vi "XML - Get relative RT Driver VI path.vi"(7 "Target Type (Windows)":T1, 10 "CD Template":refnum<class "NIVS_CD Template.lvclass">, 11 "Project Name":string) -> (3 "Relative RT Driver VI path":path)   [LabVIEW 2015, in "NIVS_Consolidated_CDW_MetaDataObj.lvclass"]
doc: "Create the relative path for the RT Driver VI inside the Configuration LLB based on the name and execution mode of the new custom device."
uses:
  NIVS_Consolidated_CDW_MetaDataObj.lvclass
  Target Type.ctl
  Template Classes/NIVS_CD Template/NIVS_CD Template.lvclass
  CD Engine lvlib.ctl
  Build Spec Engine.ctl
  Build Spec Engine.vi
  CD Engine lvlib.vi
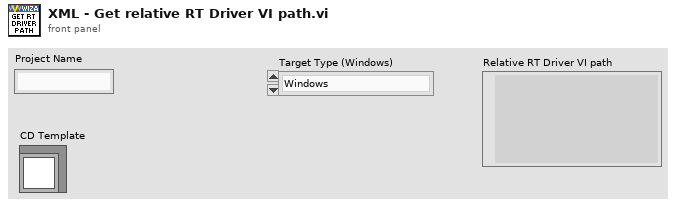
[diagram p1: front panel]
types:
  T1 = typedef "NIVS_Consolidated_CDW_MetaDataObj.lvclass/Target Type.ctl" = enum16{"Windows", "VxWorks", "Pharlap", "Linux 32 ARM", "Linux x64"}
  T2 = typedef "NIVS_Consolidated_CDW_MetaDataObj.lvclass/CD Engine lvlib.ctl" = enum16{"LibraryFileName", "LibraryFolderName", "Engine.FolderName", "Engine.Init.FolderName", "Engine.Run.FolderName", "Engine.Shutdown.FolderName", "Types.FolderName", "Engine.RT Driver VI.TemplatePath", "Engine.RT Driver VI.FileName", "Engine.RTStateVariables.Name", "Engine.RTStateVariables.Name.NoExtension", "Engine.Async.NameExtension", "Engine.Async.TemplateName"}
  T3 = typedef "NIVS_Consolidated_CDW_MetaDataObj.lvclass/Build Spec Engine.ctl" = enum16{"Destinations.LLBWindowsFileName", "Destinations.LLBVxWorksFileName", "Destinations.LLBPharlapFileName", "Destinations.LLBLinuxARMFileName", "Destinations.LLBLinux64FileName"}
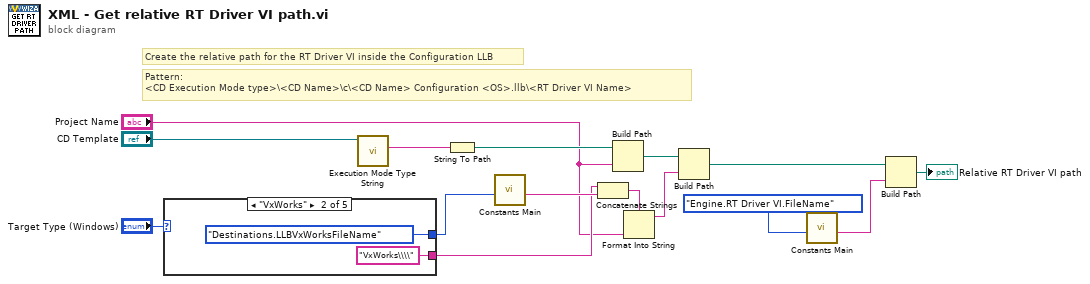
[diagram p0: block diagram]
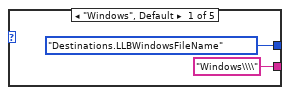
[diagram p2: hidden frame]
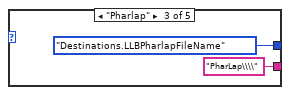
[diagram p3: hidden frame]
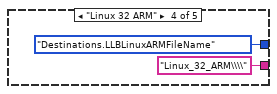
[diagram p4: hidden frame]
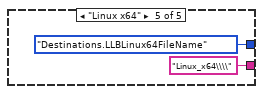
[diagram p5: hidden frame]
diagram:
  # "Create the relative path for the RT Driver VI inside the Configuration LLB"
  # "Pattern:\n<CD Execution Mode type>\\<CD Name>\\c\\<CD Name> Configuration <OS>.llb\\<RT Driver VI Name>"
  n1 = case shown="\"VxWorks\"" "Target Type (Windows)" {
    tunnel: [Build_Spec_Engine."Destinations.LLBWindowsFileName" ("Action") Build_Spec_Engine."Destinations.LLBVxWorksFileName" ("Action") Build_Spec_Engine."Destinations.LLBPharlapFileName" ("Action") Build_Spec_Engine."Destinations.LLBLinuxARMFileName" ("Action") Build_Spec_Engine."Destinations.LLBLinux64FileName" ("Action")] -> w7
    tunnel: ["Windows\\\\" ("format string") "VxWorks\\\\" ("format string") "PharLap\\\\" ("format string") "Linux_32_ARM\\\\" ("format string") "Linux_x64\\\\" ("format string")] -> w4
    frame "Windows", Default {
    }
    frame "VxWorks" {
    }
    frame "Pharlap" {
    }
    frame "Linux 32 ARM" {
    }
    frame "Linux x64" {
    }
  }
  n2 = call-dynamic "Execution Mode Type String.vi"("CD Template"="CD Template") -> ("Execution Mode Type String"=w1:string)  [unwired: 10 in]
  n3 = String To Path(string=w1) -> (path=w12:path)
  n4 = call-poly "Constants Main.vi"("Action"=w7) -> ("Output"=w6:string)  [unwired: 10 in]
  n5 = Concatenate Strings(w4, w6) -> (w5:string)
  n6 = Build Path(base path=w12, name or relative path="Project Name") -> (appended path=w11:path)
  n7 = Format Into String(format string=w5, "Project Name") -> (resulting string=w13:string)  [unwired: 2 in, 1 out]
  n8 = Build Path(base path=w11, name or relative path=w13) -> (appended path=w9:path)
  n9 = call-poly "Constants Main.vi"("Action"=CD_Engine_lvlib."Engine.RT Driver VI.FileName") -> ("Output"=w8:string)  [unwired: 10 in]
  n10 = Build Path(base path=w9, name or relative path=w8) -> (appended path=→"Relative RT Driver VI path":path)
